vi "_040.vi"() -> ()   [LabVIEW 2024]
panel:
  in  "Switch":bool
  out "Alphabets :":string
  out "ASCII":i32[](array[numeric])
  # "Generate Alphabets :"
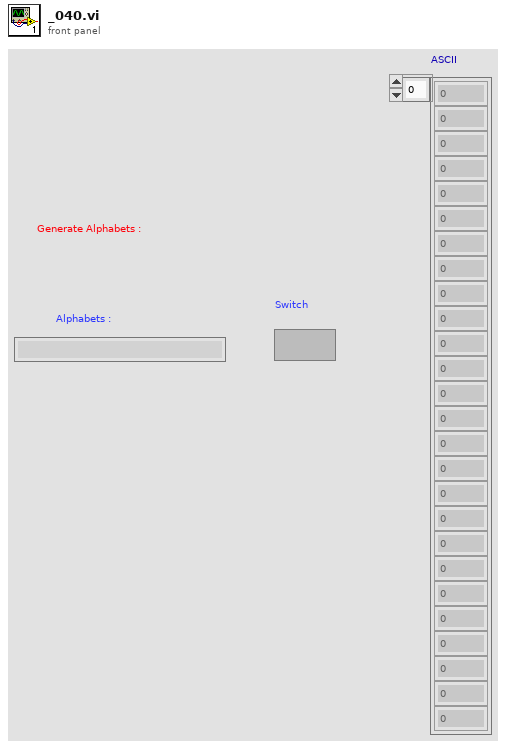
[diagram p1: front panel]
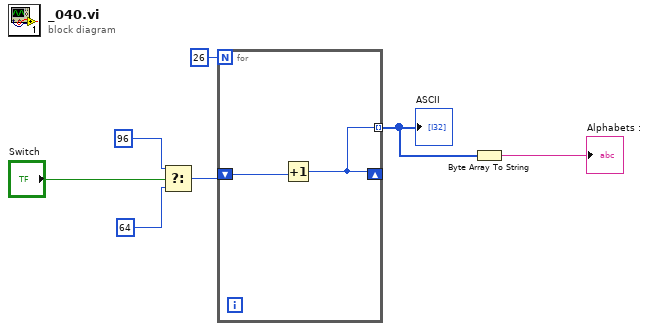
[diagram p0: block diagram]
diagram:
  n1 = Select(t=96, s="Switch", f=64) -> (s? t:f=w5:i32)
  n2 = for {
    N: 26 -> [_]
    shift-right: [w8] -> _
    shift-left: w5 -> [w9]
    tunnel: [w8] -> w3 mode=indexing
    n3 = Increment(x=w9) -> (x+1=w8:i32)
  }
  "ASCII" <- w3
  n4 = Byte Array To String(unsigned byte array=w3) -> (string=→"Alphabets :":string)
